vi "Build Probe VI.vi"(8 "error in":errorcluster, 9 "Cache Probe VI":path, 10 "VI in":refnum<vi>, 11 "Level's Data in":T1[](array[typedef])) -> (0 "error out":errorcluster)   [LabVIEW 2019, in "GOOP Probe.lvlib"]
uses:
  GOOP Probe.lvlib
  Level Data.ctl
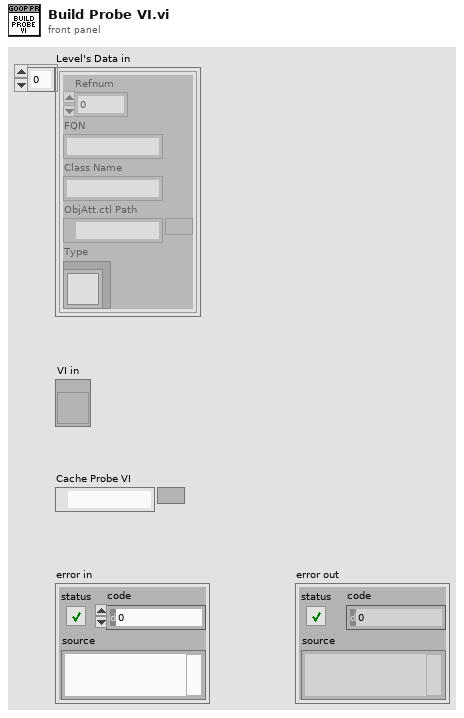
[diagram p1: front panel]
types:
  T1 = typedef "GOOP Probe.lvlib/Level Data.ctl" = cluster{"Refnum":i32, "FQN":string, "Class Name":string, "ObjAtt.ctl Path":path, "Type":refnum<class>}
  T2 = enum16{"Share clones between instances", "Preallocate clone for each instance"}
  T3 = typedef "LVPositionTypeDef.ctl" = cluster{"Left":i32, "Top":i32}
  T4 = typedef "LVRectTypeDef.ctl" = cluster{"Left":i16, "Top":i16, "Right":i16, "Bottom":i16}
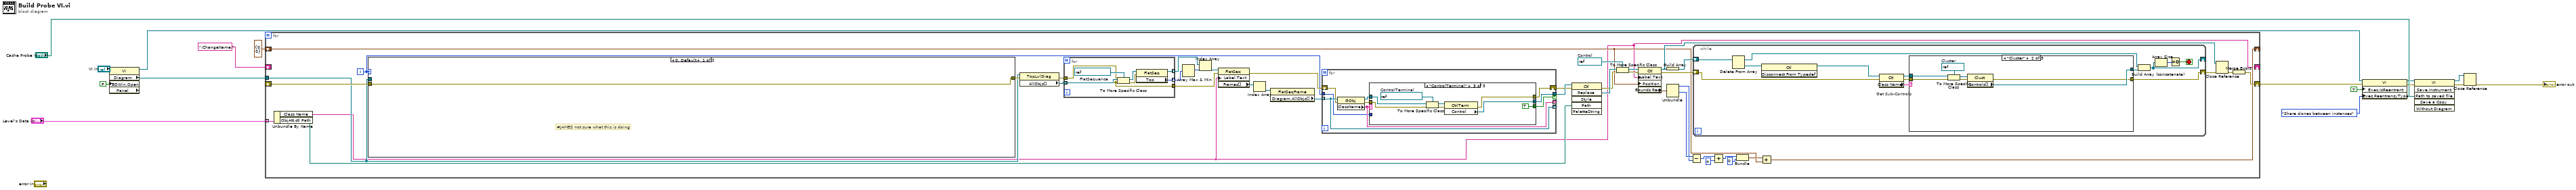
[diagram p0: block diagram]
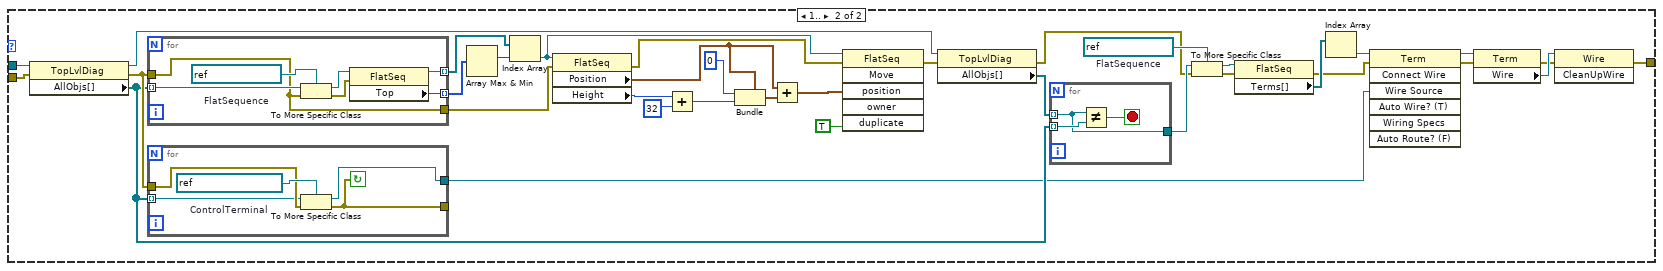
[diagram p2: hidden frame]
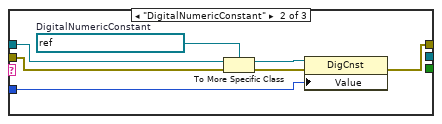
[diagram p4: hidden frame]
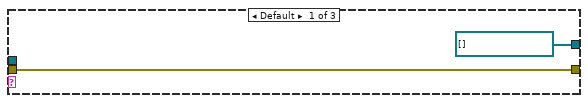
[diagram p5: hidden frame]
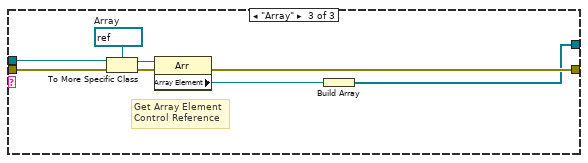
[diagram p6: hidden frame]
diagram:
  n1 = property class="VI" props=["Diagram", "BDWin.Open", "Panel"](reference="VI in", "BDWin.Open"=FALSE ("Block Diagram Window:Open")) -> (reference out=w13:refnum<vi>, "Diagram"=w5:refnum<vi>)  [unwired: 1 in, 2 out]
  n2 = for {
    tunnel: w5 -> [w39]
    shift-right: [w57] -> w10
    shift-left: _ -> [w41]
    shift-right: [w29] -> _
    shift-left: cluster{i16, "Left":i32} {0, "Left"=0} -> [w32]
    shift-right: [w17] -> _
    shift-left: ":ChangeName:" ("y") -> [_]
    tunnel: "Level's Data in" -> [w19] mode=indexing
    i -> [w42]
    w56 = refnum<vi> refnum  # Control
    n3 = Unbundle By Name(w19) -> ("Class Name"=w17:string, "ObjAtt.ctl Path"=w18:path)
    n4 = case shown="0, Default" w42 {
      tunnel: w41 -> [w65 w98]
      tunnel: [w65 w70] -> w40
      tunnel: w39 -> [_ w100]
      frame 0, Default {
        # "#JAMES not sure what this is doing"
      }
      frame 1.. {
        w85 = refnum<vi> refnum  # FlatSequence
        n5 = property class="TopLvlDiag"(reference=w100, error in=w98) -> (reference out=w87:refnum<vi>, error out=w82:errorcluster, "AllObjs[]"=w81:refnum<vi>[])
        n6 = for {
          tunnel: w81 -> [w114] mode=indexing
          tunnel: w82 -> [w111]
          tunnel: [w111] -> w97
          tunnel: [w110] -> w69 mode=indexing
          tunnel: [w109] -> w68 mode=indexing
          w115 = refnum<vi> refnum  # FlatSequence
          n7 = To More Specific Class(target class=w115, reference=w114, error in=w111) -> (specific class reference=w113:refnum<vi>, error out=w112:errorcluster)
          n8 = property class="FlatSeq"(reference=w113, error in=w112) -> (reference out=w109:refnum<vi>, "Top"=w110:i32)  [unwired: 1 out]
        }
        n9 = for {
          tunnel: [w105] -> w76
          tunnel: w81 -> [w102] mode=indexing
          tunnel: w82 -> [w103]
          tunnel: [w101] -> _
          stop <- w101 continue-if-true
          w104 = refnum<vi> refnum  # ControlTerminal
          n10 = To More Specific Class(target class=w104, reference=w102, error in=w103) -> (specific class reference=w105:refnum<vi>, error out=w101:errorcluster)
        }
        n11 = Array Max & Min(array=w69) -> (max index (indices)=w67:i32)  [unwired: 3 out]
        n12 = Index Array(array=w68, index=w67) -> (element=w66:refnum<vi>)
        n13 = property class="FlatSeq"(reference=w66, error in=w97) -> (error out=w89:errorcluster, "Position"=w94:T3, "Height"=w92:u32)  [unwired: 1 out]
        n14 = Add(x=w92, y=32 ("Left")) -> (x+y=w90:u32)
        n15 = Bundle(cluster=w94, "Left"=0, "Top"=w90) -> (w95:T3)
        n16 = Add(x=w94, y=w95) -> (x+y=w96:T3)
        n17 = invoke class="FlatSeq" method="Move"(reference=w66, error in=w89, "position"=w96, "duplicate"=TRUE ("Duplicate? (F)")) -> (error out=w88:errorcluster)  [unwired: 2 in, 5 out]
        n18 = property class="TopLvlDiag"(reference=w87, error in=w88) -> (error out=w83:errorcluster, "AllObjs[]"=w86:refnum<vi>[])  [unwired: 1 out]
        n19 = for {
          tunnel: w86 -> [w106] mode=indexing
          tunnel: w81 -> [w108] mode=indexing
          tunnel: [w106] -> w84
          stop <- w107 stop-if-true
          n20 = Not Equal?(x=w106, y=w108) -> (x != y?=w107:bool)
        }
        n21 = To More Specific Class(target class=w85, reference=w84, error in=w83) -> (specific class reference=w80:refnum<vi>, error out=w79:errorcluster)
        n22 = property class="FlatSeq"(reference=w80, error in=w79) -> (error out=w75:errorcluster, "Terms[]"=w78:refnum<vi>[])  [unwired: 1 out]
        n23 = Index Array(array=w78) -> (element=w77:refnum<vi>)  [unwired: 1 in]
        n24 = invoke class="Term" method="Connect Wire"(reference=w77, error in=w75, "Wire Source"=w76) -> (reference out=w74:refnum<vi>, error out=w73:errorcluster)  [unwired: 4 in, 5 out]
        n25 = property class="Term"(reference=w74, error in=w73) -> (error out=w71:errorcluster, "Wire"=w72:refnum<vi>)  [unwired: 1 out]
        n26 = invoke class="Wire" method="CleanUpWire"(reference=w72, error in=w71) -> (error out=w70:errorcluster)  [unwired: 1 in, 2 out]
      }
    }
    n27 = property class="TopLvlDiag"(reference=w39, error in=w40) -> (error out=w22:errorcluster, "AllObjs[]"=w25:refnum<vi>[])  [unwired: 1 out]
    n28 = for {
      tunnel: w25 -> [w63] mode=indexing
      tunnel: w22 -> [w60]
      tunnel: [w60] -> w24
      tunnel: [w59] -> w28 mode=indexing
      tunnel: [w58] -> w27 mode=indexing
      w64 = refnum<vi> refnum  # FlatSequence
      n29 = To More Specific Class(target class=w64, reference=w63, error in=w60) -> (specific class reference=w62:refnum<vi>, error out=w61:errorcluster)
      n30 = property class="FlatSeq"(reference=w62, error in=w61) -> (reference out=w58:refnum<vi>, "Top"=w59:i32)  [unwired: 1 out]
    }
    n31 = Array Max & Min(array=w28) -> (max index (indices)=w26:i32)  [unwired: 3 out]
    n32 = Index Array(array=w27, index=w26) -> (element=w23:refnum<vi>)
    n33 = property class="FlatSeq"(reference=w23, error in=w24, "Label.Text"=w17) -> (error out=w43:errorcluster, "Frames[]"=w46:refnum<vi>[])  [unwired: 1 out]
    n34 = Index Array(array=w46) -> (element=w45:refnum<vi>)  [unwired: 1 in]
    n35 = property class="FlatSeqFrame"(reference=w45) -> ("Diagram.AllObjs[]"=w44:refnum<vi>[])  [unwired: 1 in, 2 out]
    n36 = for {
      tunnel: w44 -> [w122] mode=indexing
      tunnel: [w124] -> _ mode=indexing
      tunnel: [w122] -> _ mode=indexing
      tunnel: w42 -> [w121]
      shift-right: [w118] -> w20
      shift-left: w43 -> [w120]
      tunnel: [w117] -> w21 if=w116
      n37 = property class="GObj"(reference=w122, error in=w120) -> (reference out=w123:refnum<vi>, error out=w119:errorcluster, "ClassName"=w124:string)
      n38 = case shown="\"ControlTerminal\"" w124 {
        tunnel: w123 -> [_ w132 w140]
        tunnel: w121 -> [_ w131 _]
        tunnel: w119 -> [w125 w128 w137]
        tunnel: [w125 w126 w135] -> w118
        tunnel: [_ _ w134] -> w117
        tunnel: [_ _ TRUE] -> w116
        frame Default {
        }
        frame "DigitalNumericConstant" {
          w130 = refnum<vi> refnum  # DigitalNumericConstant
          n39 = To More Specific Class(target class=w130, reference=w132, error in=w128) -> (specific class reference=w129:refnum<vi>, error out=w127:errorcluster)
          n40 = property class="DigCnst"(reference=w129, error in=w127, "Value"=w131) -> (error out=w126:errorcluster)  [unwired: 1 out]
        }
        frame "ControlTerminal" {
          w139 = refnum<vi> refnum  # ControlTerminal
          n41 = To More Specific Class(target class=w139, reference=w140, error in=w137) -> (specific class reference=w138:refnum<vi>, error out=w136:errorcluster)
          n42 = property class="CtrlTerm"(reference=w138, error in=w136) -> (error out=w135:errorcluster, "Control"=w134:refnum<vi>)  [unwired: 1 out]
        }
      }
    }
    n43 = invoke class="Ctl" method="Replace"(reference=w21, error in=w20, "Path"=w18) -> (error out=w52:errorcluster, "Replace"=w53:refnum<vi>)  [unwired: 3 in, 4 out]
    n44 = To More Specific Class(target class=w56, reference=w53, error in=w52) -> (specific class reference=w50:refnum<vi>, error out=w48:errorcluster)
    n45 = property class="Ctl"(reference=w50, error in=w48, "Label.Text"=w17, "Position"=w32) -> (reference out=w49:refnum<vi>, error out=w47:errorcluster, "Bounds Rect"=w38:T4)
    n46 = Build Array(w49) -> (w55:refnum<vi>[])
    n47 = Unbundle(w38) -> ("Left"=w36:i16, "Right"=w37:i16)  [unwired: 2 out]
    n48 = Subtract(x=w37, y=w36) -> (x-y=w35:i16)
    n49 = while {
      shift-right: [w145] -> _
      shift-left: w55 -> [w148]
      shift-right: [w149] -> w54
      shift-left: w47 -> [w141]
      stop <- w143 stop-if-true
      n50 = Delete From Array(array=w148) -> (deleted portion=w142:refnum<vi>, array with subset deleted=w147:refnum<vi>[])  [unwired: 2 in]
      n51 = invoke class="Ctl" method="Disconnect From Typedef"(reference=w142) -> (reference out=w146:refnum<vi>)  [unwired: 2 in, 2 out]
      n52 = property class="Ctl"(reference=w146, error in=w141) -> (reference out=w152:refnum<vi>, error out=w151:errorcluster, "Class Name"=w153:string)
      n53 = case "Get Sub-Controls" shown="\"Cluster\"" w153 {
        tunnel: w152 -> [_ w162 w170]
        tunnel: w151 -> [w155 w159 w167]
        tunnel: [refnum<vi>[] [] ("Controls[]") w157 w163] -> w150
        tunnel: [w155 w156 w165] -> w149
        frame Default {
        }
        frame "Cluster" {
          w160 = refnum<vi> refnum  # Cluster
          n54 = To More Specific Class(target class=w160, reference=w162, error in=w159) -> (specific class reference=w161:refnum<vi>, error out=w158:errorcluster)
          n55 = property class="Clust"(reference=w161, error in=w158) -> (error out=w156:errorcluster, "Controls[]"=w157:refnum<vi>[])  [unwired: 1 out]
        }
        frame "Array" {
          w168 = refnum<vi> refnum  # Array
          # "Get Array Element Control Reference"
          n56 = To More Specific Class(target class=w168, reference=w170, error in=w167) -> (specific class reference=w169:refnum<vi>, error out=w166:errorcluster)
          n57 = property class="Arr"(reference=w169, error in=w166) -> (error out=w165:errorcluster, "Array Element"=w164:refnum<vi>)  [unwired: 1 out]
          n58 = Build Array(w164) -> (w163:refnum<vi>[])
        }
      }
      n59 = Build Array (concatenate)(w147, w150) -> (w145:refnum<vi>[])
      n60 = Array Size(array=w145) -> (size(s)=w144:i32)
      n61 = Equal To 0?(x=w144) -> (x = 0?=w143:bool)
    }
    n62 = Add(x=w35, y=i16 4) -> (x+y=w33:i16)
    n63 = Bundle(w33, "Left"=0) -> (w31:cluster{i16, "Left":i32})  [unwired: 1 in]
    n64 = Add(x=w31, y=w32) -> (x+y=w29:cluster{i16, "Left":i32})
    n65 = Close Reference(reference=w49, error in (no error)=w54) -> (error out=w51:errorcluster)
    n66 = Merge Errors(w51) -> (w57:errorcluster)
  }
  n67 = property class="VI"(reference=w13, error in=w10, "Exec.IsReentrant"=TRUE ("Execution:Is Reentrant"), "Exec.ReentrancyType"=T2."Share clones between instances" ("Execution:Reentrancy Type")) -> (reference out=w8:refnum<vi>, error out=w7:errorcluster)
  n68 = invoke class="VI" method="Save.Instrument"(reference=w8, error in=w7, "Path to saved file"="Cache Probe VI") -> (reference out=w9:refnum<vi>, error out=w6:errorcluster)  [unwired: 3 in, 4 out]
  n69 = Close Reference(reference=w9, error in (no error)=w6) -> (error out=→"error out":errorcluster)
